vi "Append image and delete if possible.vi"(0 "report in":refnum<class "NI_report.lvclass">, 1 "alignment (default)":T1, 5 "path to image":path, 11 "error in (no error)":errorcluster, 12 "caption or alternative string":string, 13 "MS Office parameters":T2) -> (4 "report out":refnum<class "NI_report.lvclass">, 8 "start out Word)":i32, 10 "end out Word)":i32, 15 "error out":errorcluster)   [LabVIEW 2017, in "NI_report.lvclass"]
uses:
  <vilib>/Utility/NIReport.llb/NI_report.lvclass
  <vilib>/Utility/NIReport.llb/HTML Report Image Alignment.ctl
  <vilib>/Utility/NIReport.llb/NI_ReportGenerationCore.lvlib
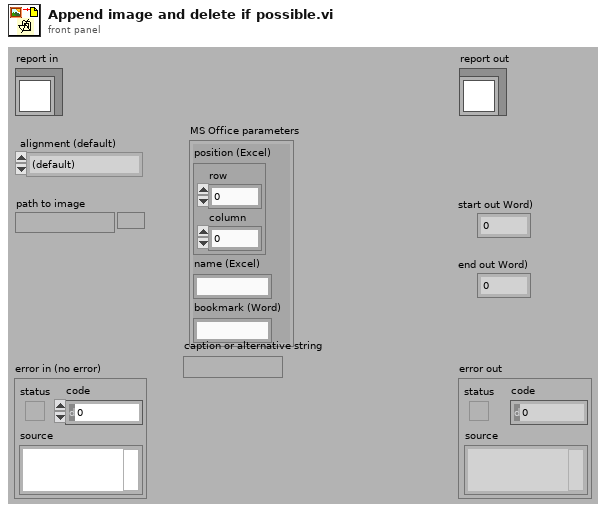
[diagram p1: front panel]
types:
  T1 = typedef "NI_ReportGenerationCore.lvlib/HTML Report Image Alignment.ctl" = enum16{"(default)", "LEFT", "RIGHT", "TOP", "TEXTTOP", "MIDDLE", "ABSMIDDLE", "BASELINE", "BOTTOM", "ABSBOTTOM"}
  T2 = cluster{"position (Excel)":cluster{"row":i32, "column":i32}, "name (Excel)":string, "bookmark (Word)":string}
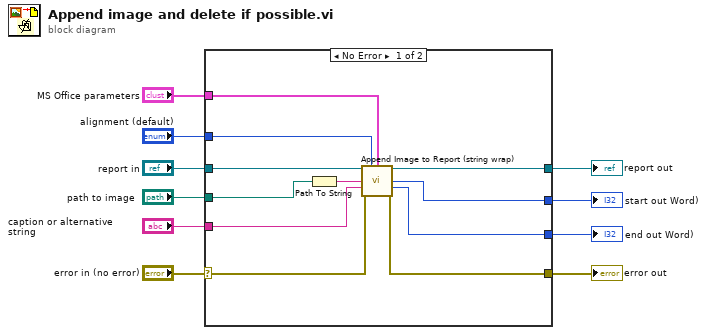
[diagram p0: block diagram]
diagram:
  n1 = case shown="No Error" "error in (no error)" {
    selector: "error in (no error)" -> [w20 w23]
    tunnel: [w13 w23] -> w9
    tunnel: [w14 w22] -> w7
    tunnel: "report in" -> [w15 w22]
    tunnel: "MS Office parameters" -> [w19 _]
    tunnel: "alignment (default)" -> [w18 _]
    tunnel: "caption or alternative string" -> [w17 _]
    tunnel: "path to image" -> [w16 _]
    tunnel: [w12 _] -> w2
    tunnel: [w11 _] -> w1
    frame No Error {
      n2 = Path To String(path=w16) -> (string=w21:string)
      n3 = call <vilib>:"Append Image to Report (string wrap).vi"("report in"=w15, "alignment (default)"=w18, "MS Office parameters"=w19, "path or URL of image"=w21, "caption or alternative string"=w17, "error in (no error)"=w20) -> ("report out"=w14:refnum<class "NI_report.lvclass">, "start out (Word)"=w12:i32, "end out (Word)"=w11:i32, "error out"=w13:errorcluster)  [unwired: 6 out]
    }
    frame Error {
    }
  }
  "error out" <- w9
  "report out" <- w7
  "start out Word)" <- w2
  "end out Word)" <- w1
